vi "Smite.vi"(8 "Error In":errorcluster) -> (0 "Error Out":errorcluster)   [LabVIEW 2017, in "Tests.lvlib"]
uses:
  Tests.lvlib
  <vilib>/addons/_JKI Toolkits/Caraya/classes/Test/Test.lvclass
  <vilib>/addons/_JKI Toolkits/Caraya/classes/Assert/Assert.lvclass
  src/Toolkit/Toolkit.lvlib
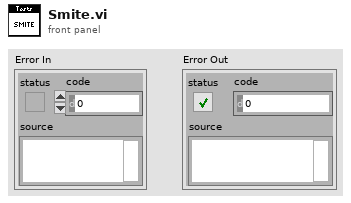
[diagram p1: front panel]
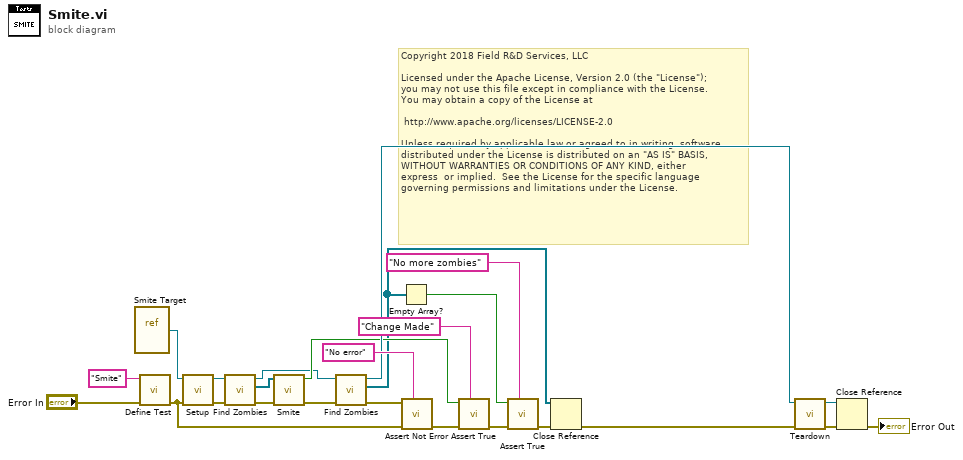
[diagram p0: block diagram]
diagram:
  # "Copyright 2018 Field R&D Services, LLC\n\nLicensed under the Apache License, Version 2.0 (the \"License\");\nyou may not use this file except in compliance with the License.\nYou may obtain a copy of the License at\n\n\thttp://www.apache.org/licenses/LICENSE-2.0\n\nUnless required by applicable law or agreed to in writing, software\ndistributed under the License is distributed on an \"AS IS\" BASIS,\nWITHOUT WARRANTIES OR CONDITIONS OF ANY KIND, either \nexpress  or implied.  See the License for the specific language \ngoverning permissions and limitations under the License."
  n1 = vi-ref "Smite Target.vi"() -> (w9:refnum<vi>)
  n2 = call <vilib>:"Define Test.vi"("error in (no error)"="Error In", "Label (VI Title)"="Smite") -> ("error out"=w5:errorcluster)  [unwired: 9 in]
  n3 = call "Setup.vi"("Error In"=w5, "VI In"=w9) -> ("Error Out"=w4:errorcluster, "VI Out"=w6:refnum<vi>)  [unwired: 8 in]
  n4 = call "Find Zombies.vi"("Error In"=w4, "VI In"=w6) -> ("Error Out"=w12:errorcluster, "Graves"=w10:refnum<vi>[], "VI Out"=w11:refnum<vi>)  [unwired: 7 in]
  n5 = call "Smite.vi"("Error In"=w12, "Graves"=w10) -> ("Error Out"=w25:errorcluster, "Change Made?"=w14:bool)  [unwired: 8 in]
  n6 = call "Find Zombies.vi"("Error In"=w25, "VI In"=w11) -> ("Error Out"=w20:errorcluster, "Graves"=w7:refnum<vi>[], "VI Out"=w17:refnum<vi>)  [unwired: 7 in]
  n7 = Empty Array?(array=w7) -> (empty?=w8:bool)
  n8 = call <vilib>:"Assert Not Error.vi"("Label"="No error", "error in (no error)"=w5, "Not Error?"=w20) -> ("error out"=w22:errorcluster)  [unwired: 8 in]
  n9 = call <vilib>:"Assert True.vi"("Label"="Change Made", "error in (no error)"=w22, "True?"=w14) -> ("error out"=w15:errorcluster)  [unwired: 8 in]
  n10 = call <vilib>:"Assert True.vi"("Label"="No more zombies", "error in (no error)"=w15, "True?"=w8) -> ("error out"=w18:errorcluster)  [unwired: 8 in]
  n11 = Close Reference(reference=w7, error in (no error)=w18) -> (error out=w2:errorcluster)
  n12 = call "Teardown.vi"("Error In"=w2, "VI In"=w17) -> ("Error Out"=w1:errorcluster, "VI Out"=w3:refnum<vi>)  [unwired: 8 in]
  n13 = Close Reference(reference=w3, error in (no error)=w1) -> (error out=→"Error Out":errorcluster)
